vi "temp_hygro(mock).vi"() -> (2 "temp":string, 3 "humidity":string)   [LabVIEW 2013, in "TempHygro.lvlib"]
uses:
  lib/TempHygro.lvlib
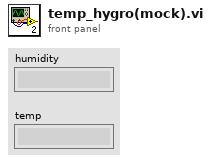
[diagram p1: front panel]
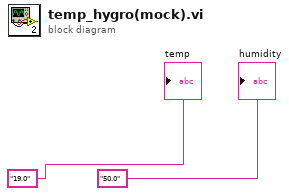
[diagram p0: block diagram]
diagram:
  "humidity" <- "50.0"
  "temp" <- "19.0"
